vi "Bulk Mode Read Data.vi"(7 "SlaveID":u8=1, 8 "error in (no error)":errorcluster, 9 "# samples to read":u16, 11 ".NET Refnum in":refnum<k24>) -> (0 "error out":errorcluster, 1 "# samples in buffer":u16, 2 "Vib":u16[](array[numeric]), 3 "reference out":refnum<k24>)   [LabVIEW 2017]
uses:
  dll/Modbus.dll
panel:
  out "-1 = Normal Mode":i16
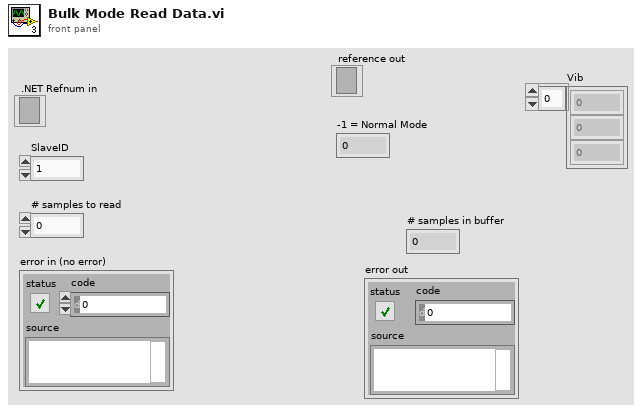
[diagram p1: front panel]
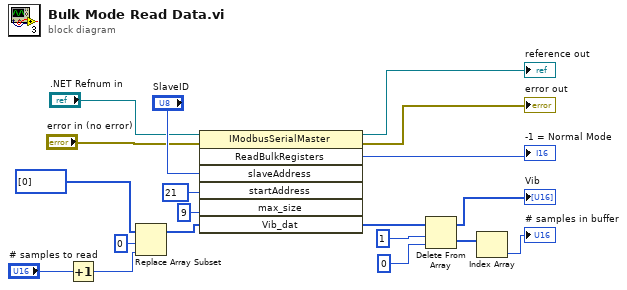
[diagram p0: block diagram]
diagram:
  n1 = Increment(x="# samples to read") -> (x+1=w9:u16)
  n2 = Replace Array Subset(array=u16[] [0], new element=w9, index=0) -> (w6:u16[])
  n3 = invoke class="IModbusSerialMaster" method="ReadBulkRegisters"(reference=".NET Refnum in", error in="error in (no error)", "slaveAddress"="SlaveID", "startAddress"=u16 21, "max_size"=i16 9, "Vib_dat"=w6) -> (reference out=→"reference out":refnum<k24>, error out=→"error out":errorcluster, "ReadBulkRegisters"=→"-1 = Normal Mode":i16, "Vib_dat"=w5:u16[])  [unwired: 1 in, 3 out]
  n4 = Delete From Array(array=w5, length=1, index=0) -> (deleted portion=w4:u16[], array with subset deleted=→"Vib":u16[])
  n5 = Index Array(array=w4) -> (element=→"# samples in buffer":u16)  [unwired: 1 in]
